vi "Command with Response Check.vi"(8 "error in (no error)":errorcluster, 10 "Data":string, 11 "TCP Network Connection in":refnum<k5>) -> (0 "error out":errorcluster, 1 "Returned String":string, 2 "Returned Error":bool, 3 "TCP Network Connection out":refnum<k5>)   [LabVIEW 2020]
doc: "Author: Scott Hannahs <sth@magnet.fsu.edu>\nCopyright 2018 Florida State University, All rights reserved."
uses:
  Interlock 32T Net Client Globals.vi
  <vilib>/regexp/Match Regular Expression.xnode
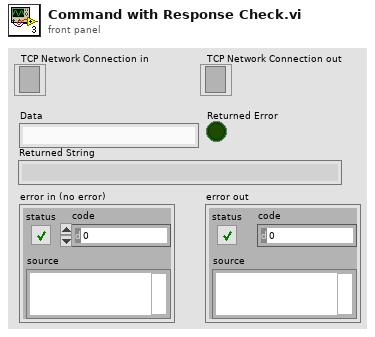
[diagram p1: front panel]
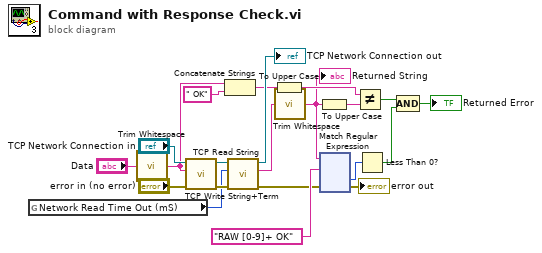
[diagram p0: block diagram]
diagram:
  n1 = global read "Interlock 32T Net Client Globals.vi" "Network Read Time Out (mS)"() -> (w1:i32)
  n2 = call <vilib>:"Trim Whitespace.vi"("string"="Data") -> ("trimmed string"=w7:string)  [unwired: 1 in]
  n3 = call "TCP Write String+Term.vi"("Error In"="error in (no error)", "Data"=w7, "connection ID"="TCP Network Connection in") -> ("Error Out"=w3:errorcluster, "connection ID out"=w19:refnum<k5>)  [unwired: 7 in]
  n4 = Concatenate Strings(w7, " OK" ("string")) -> (w14:string)
  n5 = call "TCP Read String.vi"("Error In"=w3, "timeout ms (1000)"=w1, "TCP Network Connection in"=w19) -> ("Error Out"=w4:errorcluster, "String"=w11:string, "TCP Network Connection out"=→"TCP Network Connection out":refnum<k5>)  [unwired: 6 in]
  n6 = To Upper Case(1:w14) -> (0:w13:string)
  n7 = call <vilib>:"Trim Whitespace.vi"("string"=w11) -> ("trimmed string"=w2:string)  [unwired: 1 in]
  "Returned String" <- w2
  n8 = To Upper Case(1:w2) -> (0:w6:string)
  n9 = xnode "Match Regular Expression"("input string"=w2, "regular expression"="RAW [0-9]+ OK", "error in"=w4) -> ("offset past match"=w9:i32, "error out"=→"error out":errorcluster)  [unwired: 3 in, 3 out]
  n10 = Not Equal?(x=w13, y=w6) -> (x != y?=w16:bool)
  n11 = Less Than 0?(x=w9) -> (x < 0?=w8:bool)
  n12 = Compound Arithmetic op=AND(w16, w8) -> (→"Returned Error":bool)
